vi "initialise.vi"(8 "error in (no error)":errorcluster, 11 "GenericPlugin in":refnum<class "LightSourceMH110125Tsunami.lvclass">) -> (0 "error out":errorcluster, 3 "GenericPlugin out":refnum<class "LightSourceMH110125Tsunami.lvclass">)   [LabVIEW 2010, in "LightSourceMH110125Tsunami.lvclass"]
doc: "The dynamic dispatch-version of this VI initalises the plug-in object by allocating and initalising any dynamic resources need."
uses:
  LightSourceMH110125Tsunami.lvclass
  LightSourceScaffold/LightSourceScaffold/LightSourceScaffold.lvclass
  LightSourceMH110125Tsunami.lvclass/LightSourceMH110125Tsunami.ctl
  <vilib>/Instr/_visa.llb/VISA Configure Serial Port (Instr).vi
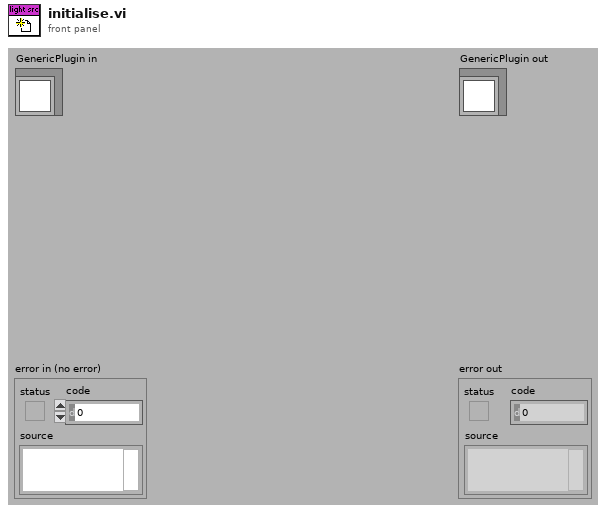
[diagram p1: front panel]
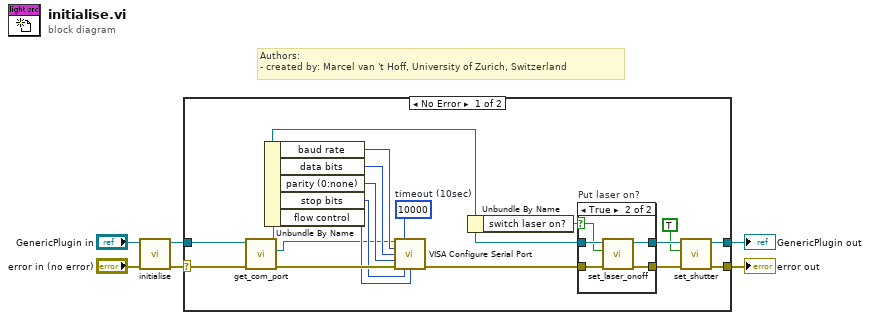
[diagram p0: block diagram]
diagram:
  # "Authors: \n- created by: Marcel van 't Hoff, University of Zurich, Switzerland"
  n1 = call-parent "initialise.vi"("error in (no error)"="error in (no error)", "GenericPlugin in"="GenericPlugin in") -> ("error out"=w4:errorcluster, "GenericPlugin out"=w2:refnum<class "LightSourceMH110125Tsunami.lvclass">)  [unwired: 8 in]
  n2 = case shown="No Error" w4 {
    selector: w4 -> [w24 w33]
    tunnel: [w8 w33] -> w3
    tunnel: w2 -> [w23 w32]
    tunnel: [w9 w32] -> w1
    frame No Error {
      w22 = u32 10000  # timeout (10sec)
      n3 = call-dynamic "get_com_port.vi"("error in (no error)"=w24, "LightSourceMH110125Tsunami in"=w23) -> ("error out"=w18:errorcluster, "comm port"=w15:refnum<visa-resource-name>, "LightSourceMH110125Tsunami out"=w12:refnum<class "LightSourceMH110125Tsunami.lvclass">)  [unwired: 7 in]
      n4 = Unbundle By Name(w12) -> ("baud rate"=w21:u32, "data bits"=w20:u16, "parity (0:none)"=w19:enum16{"None", "Odd", "Even", "Mark", "Space"}, "stop bits"=w17:u16, "flow control"=w16:u16)
      n5 = call-poly "VISA Configure Serial Port"("VISA resource name"=w15, "timeout (10sec)"=w22, "baud rate (9600)"=w21, "data bits (8)"=w20, "parity (0:none)"=w19, "error in (no error)"=w18, "stop bits (10: 1 bit)"=w17, "flow control (0:none)"=w16) -> ("error out"=w14:errorcluster)  [unwired: 1 in, 6 out]
      n6 = Unbundle By Name(w12) -> ("switch laser on?"=w13:bool)
      n7 = case "Put laser on?" shown="True" w13 {
        selector: w13 -> [_ w29]
        tunnel: w14 -> [w25 w31]
        tunnel: w12 -> [w26 w30]
        tunnel: [w25 w28] -> w11
        tunnel: [w26 w27] -> w10
        frame False {
        }
        frame True {
          n8 = call-dynamic "set_laser_onoff.vi"("error in (no error)"=w31, "on?"=w29, "LightSourceMH110125Tsunami in"=w30) -> ("error out"=w28:errorcluster, "LightSourceMH110125Tsunami out"=w27:refnum<class "LightSourceMH110125Tsunami.lvclass">)  [unwired: 7 in]
        }
      }
      n9 = call-dynamic "set_shutter.vi"("error in (no error)"=w11, "shutter open?"=TRUE, "LightSourceMH110125Tsunami in"=w10) -> ("error out"=w8:errorcluster, "LightSourceMH110125Tsunami out"=w9:refnum<class "LightSourceMH110125Tsunami.lvclass">)  [unwired: 6 in, 1 out]
    }
    frame Error {
    }
  }
  "error out" <- w3
  "GenericPlugin out" <- w1
